vi "Resolve Pin Groups to Pins.vi"(10 "group mappings":T1, 11 "pin or group names":string[](array[string])) -> (3 "resolved pin or relay names":string[](array[string]))   [LabVIEW 2020, in "NI Session Management V1 Client.lvlib" / "Session Reservation.lvclass"]
doc: "If a given pin or relay name is a group name then resolve them to pins and append them."
uses:
  Session Reservation.lvclass
  Group Mapping.ctl
  41dee1a7-95a6-4112-bccc-97afb29f1749.vi
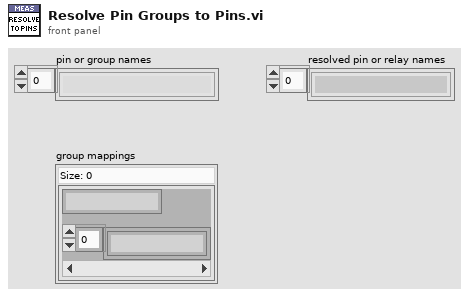
[diagram p1: front panel]
types:
  T1 = typedef "NI Session Management V1 Client.lvlib/Session Reservation.lvclass/Group Mapping.ctl" = map{string, string[]}
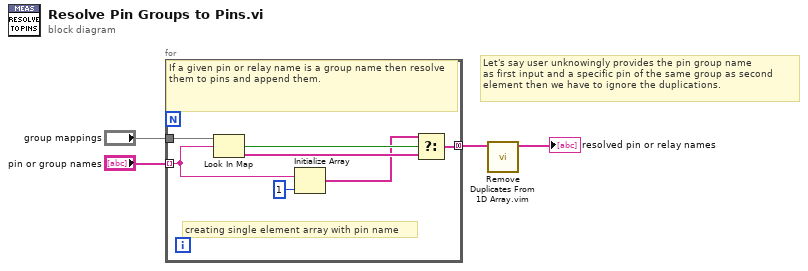
[diagram p0: block diagram]
diagram:
  # "Let's say user unknowingly provides the pin group name \nas first input and a specific pin of the same group as second\nelement then we have to ignore the duplications."
  n1 = for {
    tunnel: "pin or group names" -> [w7] mode=indexing
    tunnel: "group mappings" -> [w11]
    tunnel: [w9] -> w2 mode=concatenating
    # "creating single element array with pin name"
    # "If a given pin or relay name is a group name then resolve them to pins and append them."
    n2 = Look In Map(map=w11, key=w7) -> (key not found?=w10:bool, value=w8:string[])  [unwired: 1 in]
    n3 = Initialize Array(w7, 1 ("dimension size")) -> (w5:string[])
    n4 = Select(t=w5, s=w10, f=w8) -> (s? t:f=w9:string[])
  }
  n5 = call "Remove Duplicates From 1D Array.vim"("array"=w2) -> ("array with duplicates removed"=→"resolved pin or relay names":string[])  [unwired: 10 in]
